vi "name parser.vi"(10 "String":string) -> (1 "Valid?":bool, 2 "Parsed String":string)   [LabVIEW 2025]
panel:
  # "allowed words with any character in:\nA..Z, 0..9, -"
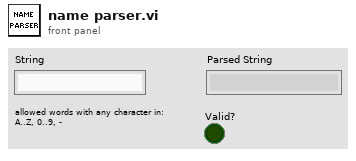
[diagram p1: front panel]
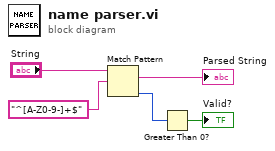
[diagram p0: block diagram]
diagram:
  n1 = Match Pattern(string="String", regular expression="^[A-Z0-9-]+$") -> (match substring=→"Parsed String":string, offset past match=w2:i32)  [unwired: 1 in, 2 out]
  n2 = Greater Than 0?(x=w2) -> (x > 0?=→"Valid?":bool)
